vi "solar_excel File Write (Append Row).vi"(6 "Visible? (F)":bool, 7 "Worksheet":string, 8 "error in (no error)":errorcluster, 10 "Row to Append":string[](array[string]), 11 "Excel Workbook (*.xlsx)":path) -> (0 "error out":errorcluster, 3 "dup Excel Workbook":path)   [LabVIEW 2018]
doc: "This appends a row the specified Excel Workbook (*.xlsx)."
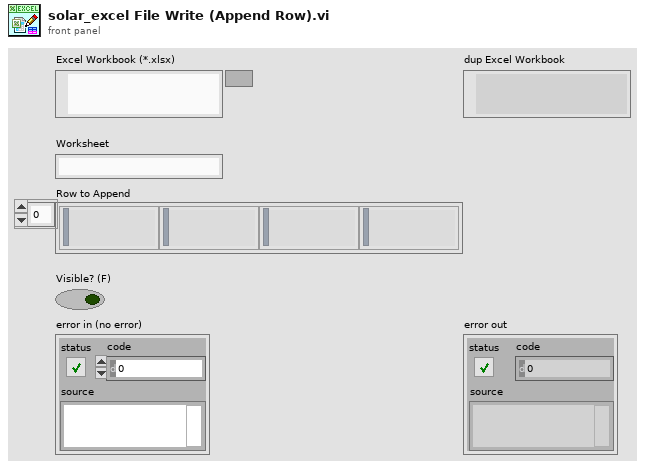
[diagram p1: front panel]
types:
  T1 = typedef "solar_excel_ctl App.ctl" = cluster{"ExcelApp":refnum<k7>, "Workbooks":refnum<k7>, "TSV":refnum<queue>}
  T2 = typedef "solar_excel_ctl Workbook.ctl" = cluster{"ExcelApp":refnum<k7>, "Workbooks":refnum<k7>, "TSV":refnum<queue>, "OpenWkb":refnum<k7>}
  T3 = typedef "solar_excel_ctl Worksheet.ctl" = cluster{"ExcelApp":refnum<k7>, "Workbooks":refnum<k7>, "TSV":refnum<queue>, "OpenWkb":refnum<k7>, "Worksheets":refnum<k7>, "OpenWksh":refnum<k7>}
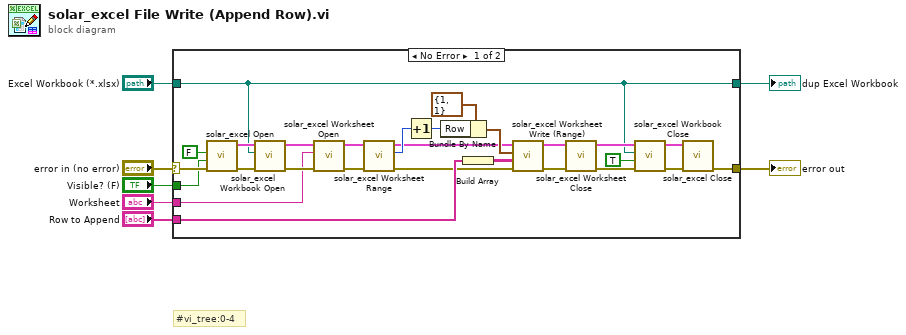
[diagram p0: block diagram]
diagram:
  # "#vi_tree:0-4"
  n1 = case shown="No Error" "error in (no error)" {
    selector: "error in (no error)" -> [w27 w36]
    tunnel: [w28 w36] -> w7
    tunnel: "Visible? (F)" -> [w26 _]
    tunnel: "Excel Workbook (*.xlsx)" -> [w20 w35]
    tunnel: "Worksheet" -> [w21 _]
    tunnel: [w20 w35] -> w2
    tunnel: "Row to Append" -> [w17 _]
    frame No Error {
      n2 = call "solar_excel Open.vi"("error in (no error)"=w27, "Visible? (F)"=w26, "Open New Instance? (F)"=FALSE) -> ("error out"=w33:errorcluster, "Excel App"=w34:T1)  [unwired: 7 in]
      n3 = call "solar_excel Workbook Open.vi"("error in (no error)"=w33, "Excel Workbook (*.xlsx)"=w20, "Excel App"=w34) -> ("error out"=w22:errorcluster, "Excel Workbook"=w23:T2)  [unwired: 7 in]
      n4 = call "solar_excel Worksheet Open.vi"("error in (no error)"=w22, "Sheet Name (STR) or Number (I32)"=w21, "Excel Workbook"=w23) -> ("error out"=w16:errorcluster, "Excel Worksheet"=w15:T3)  [unwired: 5 in, 2 out]
      n5 = call "solar_excel Worksheet Range.vi"("error in (no error)"=w16, "Excel Worksheet in"=w15) -> ("error out"=w9:errorcluster, "Rows"=w12:u32, "Excel Worksheet out"=w10:T3)  [unwired: 6 in, 1 out]
      n6 = Increment(x=w12) -> (x+1=w11:u32)
      n7 = Bundle By Name(cluster=cluster{"Row":u32, "Column":u32} {"Row"=1, "Column"=1} ("Start (1,1 = 'A1')"), "Row"=w11) -> (w13:cluster{"Row":u32, "Column":u32})
      n8 = Build Array(w17) -> (w8:string[][])
      n9 = call "solar_excel Worksheet Write (Range).vi"("error in (no error)"=w9, "Cells"=w8, "Start (1,1 = 'A1')"=w13, "Excel Worksheet in"=w10) -> ("error out"=w19:errorcluster, "Excel Worksheet out"=w18:T3)  [unwired: 6 in]
      n10 = call "solar_excel Worksheet Close.vi"("error in (no error)"=w19, "Excel Worksheet"=w18) -> ("error out"=w32:errorcluster, "Excel Workbook"=w31:T2)  [unwired: 8 in]
      n11 = call "solar_excel Workbook Close.vi"("error in (no error)"=w32, "Save? (F)"=TRUE, "Excel Workbook (*.xlsx)"=w20, "Excel Workbook"=w31) -> ("error out"=w30:errorcluster, "Excel App"=w29:T1)  [unwired: 6 in]
      n12 = call "solar_excel Close.vi"("error in (no error)"=w30, "Excel App"=w29) -> ("error out"=w28:errorcluster)  [unwired: 9 in]
    }
    frame Error {
    }
  }
  "error out" <- w7
  "dup Excel Workbook" <- w2
